vi "DetectOS.vi"() -> (3 "XP?":bool)   [LabVIEW 2012]
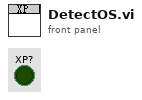
[diagram p1: front panel]
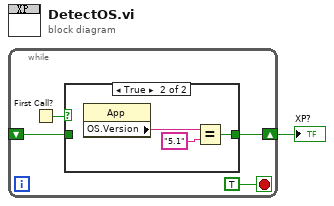
[diagram p0: block diagram]
diagram:
  n1 = while {
    shift-right: [w4] -> w1
    shift-left: _ -> [w3]
    stop <- TRUE stop-if-true
    n2 = First Call?() -> (First Call?: T/F=w5:bool)
    n3 = case shown="True" w5 {
      tunnel: [w6 w7] -> w4
      tunnel: w3 -> [w6 _]
      frame False {
      }
      frame True {
        n4 = property class="App"() -> ("OS.Version"=w9:string)  [unwired: 2 in, 2 out]
        n5 = Equal?(x=w9, y="5.1" ("Operating System:Version Number")) -> (x = y?=w7:bool)
      }
    }
  }
  "XP?" <- w1
